vi "command_file__errors.vi"() -> ()   [LabVIEW 2016]
uses:
  Instrument_Setup.vi
  Global Variables/global.vi
panel:
  in  "fehler":bool
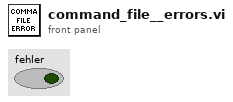
[diagram p1: front panel]
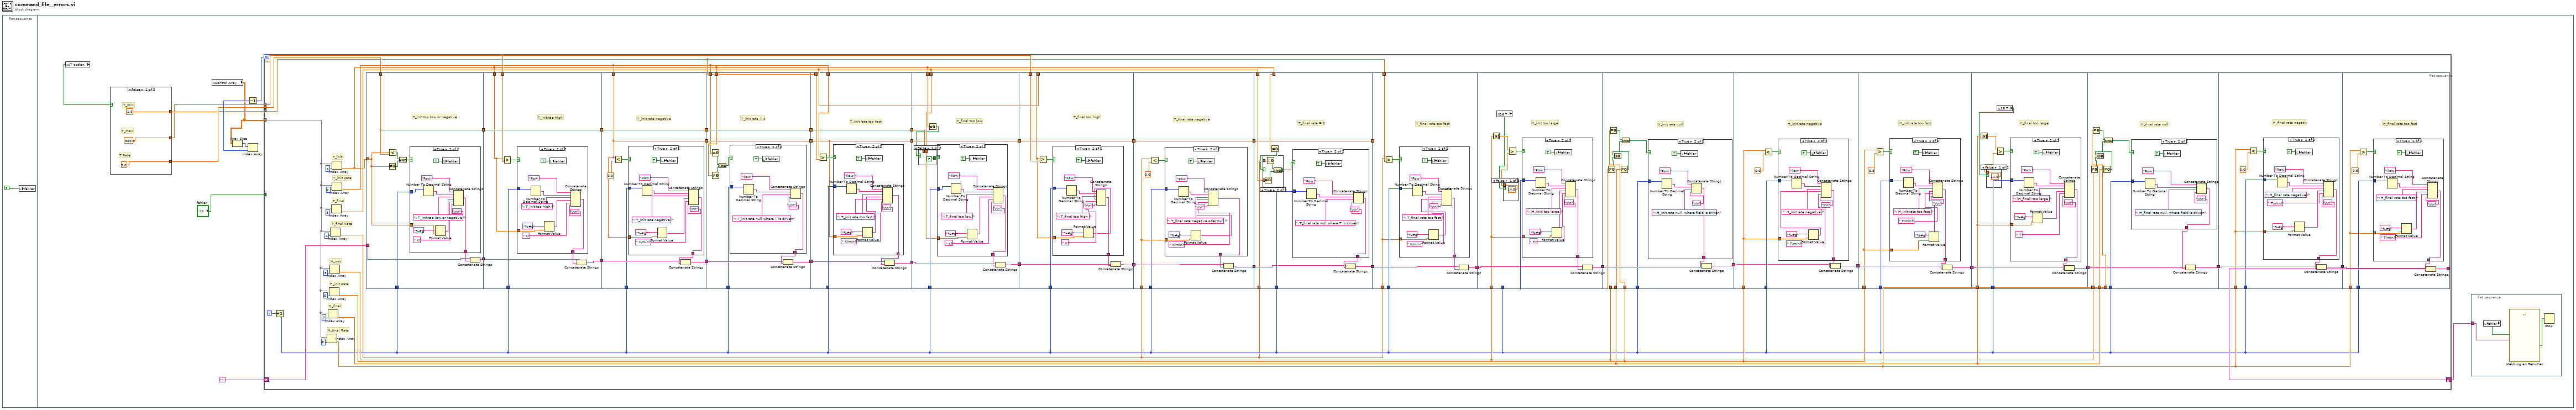
[diagram p0: block diagram]
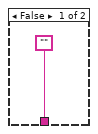
[diagram p2: hidden frame]
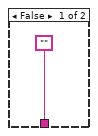
[diagram p3: hidden frame]
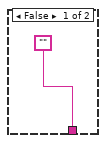
[diagram p4: hidden frame]
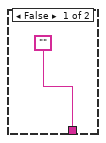
[diagram p5: hidden frame]
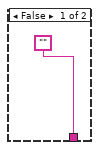
[diagram p6: hidden frame]
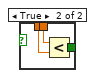
[diagram p7: hidden frame]
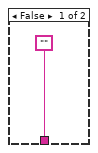
[diagram p8: hidden frame]
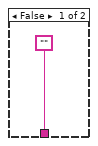
[diagram p9: hidden frame]
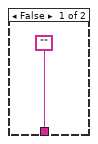
[diagram p10: hidden frame]
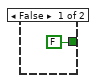
[diagram p11: hidden frame]
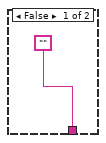
[diagram p12: hidden frame]
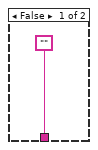
[diagram p13: hidden frame]
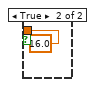
[diagram p14: hidden frame]
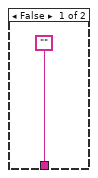
[diagram p15: hidden frame]
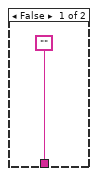
[diagram p16: hidden frame]
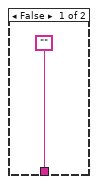
[diagram p17: hidden frame]
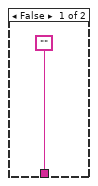
[diagram p18: hidden frame]
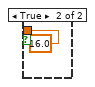
[diagram p19: hidden frame]
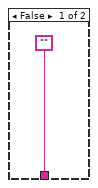
[diagram p20: hidden frame]
diagram:
  n1 = flat-sequence {
    frame #0 {
      n2 = local write "fehler"(FALSE) -> ()
    }
    frame #1 {
      n3 = global read "Instrument_Setup.vi" "JT option"() -> (w12:bool)
      n4 = case shown="False" w12 {
        tunnel: [1.6 0.02] -> w8
        tunnel: [300.0 15.0] -> w7
        tunnel: [3.0 1.0] -> w6
        frame False {
          # "T Rate"
          # "T_max"
          # "T_min"
        }
        frame True {
          # "T Rate"
          # "T_max"
          # "T_min"
        }
      }
      n5 = global read "global.vi" "Control Array"() -> (w2:dbl[][])
      n6 = Array Size(array=w2) -> (size(s)=w11:i32[])
      n7 = Index Array(array=w11) -> (element=w9:i32)  [unwired: 1 in]
      n8 = Decrement(x=w9) -> (x-1=w10:i32)
      n9 = for {
        N: w10 -> [_]
        tunnel: w2 -> [w60] mode=indexing
        tunnel: w8 -> [w59]
        tunnel: "fehler" -> [_]
        tunnel: w7 -> [w43]
        shift-right: [w35] -> w3
        shift-left: "" -> [w54]
        tunnel: w6 -> [w31]
        i -> [w57]
        # "H_final Rate"
        # "H_final"
        # "H_init Rate"
        # "H_init"
        # "T_final Rate"
        # "T_final"
        # "T_init Rate"
        # "T_init"
        n10 = Increment(x=w57) -> (x+1=w19:i32)
        n11 = Index Array(array=w60, index=8) -> (element=w32:dbl)
        n12 = Index Array(array=w60, index=7) -> (element=w34:dbl)
        n13 = Index Array(array=w60, index=6) -> (element=w40:dbl)
        n14 = Index Array(array=w60, index=5) -> (element=w33:dbl)
        n15 = Index Array(array=w60, index=4) -> (element=w18:dbl)
        n16 = Index Array(array=w60, index=3) -> (element=w17:dbl)
        n17 = Index Array(array=w60, index=1) -> (element=w16:dbl)
        n18 = Index Array(array=w60, index=2) -> (element=w20:dbl)
        n19 = flat-sequence {
          tunnel: w16 -> [w69]
          tunnel: w59 -> [w73]
          tunnel: w54 -> [w76]
          tunnel: [w75] -> w58
          tunnel: w19 -> [w74]
          tunnel: [w73] -> w47
          tunnel: w43 -> [w96]
          tunnel: w16 -> [w90]
          tunnel: w19 -> [w95]
          tunnel: w58 -> [w94]
          tunnel: [w92] -> w56
          tunnel: [w91] -> w48
          tunnel: w47 -> [w91]
          tunnel: w56 -> [w115]
          tunnel: w20 -> [w110]
          tunnel: w19 -> [w111]
          tunnel: [w113] -> w30
          tunnel: [w112] -> w28
          tunnel: w48 -> [w112]
          tunnel: [w110] -> w26
          tunnel: w30 -> [w136]
          tunnel: [w137] -> w29
          tunnel: w28 -> [w140]
          tunnel: [w140] -> w27
          tunnel: w26 -> [w139]
          tunnel: [w139] -> w25
          tunnel: w19 -> [w135]
          tunnel: w20 -> [w130]
          tunnel: w16 -> [w131]
          tunnel: [w154] -> w55
          tunnel: w20 -> [w151]
          tunnel: w19 -> [w156]
          tunnel: w29 -> [w155]
          tunnel: w31 -> [w152]
          tunnel: [w150] -> w49
          tunnel: w27 -> [w150]
          tunnel: [w149] -> w44
          tunnel: w25 -> [w149]
          tunnel: w55 -> [w177]
          tunnel: w19 -> [w178]
          tunnel: [w175] -> w53
          tunnel: w17 -> [w172]
          tunnel: w49 -> [w174]
          tunnel: [w173] -> w45
          tunnel: w44 -> [w173]
          tunnel: w16 -> [w171]
          tunnel: w19 -> [w202]
          tunnel: w53 -> [w201]
          tunnel: [w199] -> w52
          tunnel: [w198] -> w46
          tunnel: w45 -> [w198]
          tunnel: w17 -> [w196]
          tunnel: w43 -> [w197]
          tunnel: w19 -> [w222]
          tunnel: w52 -> [w221]
          tunnel: [w219] -> w24
          tunnel: w18 -> [w216]
          tunnel: [w217] -> w22
          tunnel: w46 -> [w217]
          tunnel: w24 -> [w241]
          tunnel: [w242] -> w23
          tunnel: w22 -> [w245]
          tunnel: [w245] -> w21
          tunnel: w19 -> [w243]
          tunnel: w18 -> [w240]
          tunnel: w17 -> [w239]
          tunnel: w16 -> [w238]
          tunnel: [w262] -> w51
          tunnel: w19 -> [w265]
          tunnel: w23 -> [w264]
          tunnel: w18 -> [w260]
          tunnel: w21 -> [_]
          tunnel: w31 -> [w261]
          tunnel: w51 -> [w284]
          tunnel: [w283] -> w50
          tunnel: w33 -> [w281]
          tunnel: w19 -> [w285]
          tunnel: w50 -> [w312]
          tunnel: [w311] -> w42
          tunnel: w19 -> [w310]
          tunnel: w33 -> [w309]
          tunnel: w34 -> [w308]
          tunnel: w40 -> [w302]
          tunnel: w42 -> [w324]
          tunnel: w19 -> [w325]
          tunnel: [w323] -> w41
          tunnel: w40 -> [w322]
          tunnel: [w342] -> w39
          tunnel: w19 -> [w344]
          tunnel: w41 -> [w343]
          tunnel: w40 -> [w341]
          tunnel: w39 -> [w364]
          tunnel: [w363] -> w38
          tunnel: w34 -> [w362]
          tunnel: w19 -> [w365]
          tunnel: w38 -> [w384]
          tunnel: [w383] -> w37
          tunnel: w19 -> [w388]
          tunnel: w34 -> [w387]
          tunnel: w33 -> [w386]
          tunnel: w32 -> [w385]
          tunnel: w37 -> [w405]
          tunnel: w19 -> [w406]
          tunnel: [w404] -> w36
          tunnel: w32 -> [w403]
          tunnel: [w424] -> w35
          tunnel: w36 -> [w425]
          tunnel: w19 -> [w423]
          tunnel: w32 -> [w422]
          frame #0 {
            # "T_init too low or negative"
            n20 = Not Equal To 0?(x=w69) -> (x != 0?=w72:bool)
            n21 = Less?(x=w69, y=w73) -> (x < y?=w71:bool)
            n22 = And(x=w71, y=w72) -> (x .and. y?=w70:bool)
            n23 = case shown="True" w70 {
              tunnel: w74 -> [_ w86]
              tunnel: ["" w84] -> w77
              tunnel: w69 -> [_ w81]
              frame False {
              }
              frame True {
                n24 = Number To Decimal String(number=w86) -> (decimal integer string=w85:string)  [unwired: 1 in]
                n25 = Format Value(format string="%#g", value (0)=w81) -> (output string=w79:string)  [unwired: 1 in]
                n26 = local write "fehler"(TRUE) -> ()
                n27 = Concatenate Strings("Row ", w85, ": T_init too low or negative (", w79, " K)", "\r\n") -> (w84:string)
              }
            }
            n28 = Concatenate Strings(w76, w77) -> (w75:string)
          }
          frame #1 {
            # "T_init too high"
            n29 = Greater?(x=w90, y=w96) -> (0:w97:bool)
            n30 = case shown="True" w97 {
              tunnel: ["" w105] -> w93
              tunnel: w95 -> [_ w104]
              tunnel: w90 -> [_ w99]
              frame False {
              }
              frame True {
                n31 = Number To Decimal String(number=w104) -> (decimal integer string=w106:string)  [unwired: 1 in]
                n32 = Format Value(format string="%#g", value (0)=w99) -> (output string=w101:string)  [unwired: 1 in]
                n33 = local write "fehler"(TRUE) -> ()
                n34 = Concatenate Strings("Row ", w106, ": T_init too high (", w101, " K)", "\r\n") -> (w105:string)
              }
            }
            n35 = Concatenate Strings(w94, w93) -> (w92:string)
          }
          frame #2 {
            # "T_init rate negative"
            n36 = Less?(x=w110, y=0.0) -> (x < y?=w117:bool)
            n37 = case shown="True" w117 {
              tunnel: ["" w125] -> w114
              tunnel: w111 -> [_ w124]
              tunnel: w110 -> [_ w119]
              frame False {
              }
              frame True {
                n38 = Number To Decimal String(number=w124) -> (decimal integer string=w126:string)  [unwired: 1 in]
                n39 = Format Value(format string="%#g", value (0)=w119) -> (output string=w120:string)  [unwired: 1 in]
                n40 = local write "fehler"(TRUE) -> ()
                n41 = Concatenate Strings("Row ", w126, ": T_init rate negative (", w120, " K/min)", "\r\n") -> (w125:string)
              }
            }
            n42 = Concatenate Strings(w115, w114) -> (w113:string)
          }
          frame #3 {
            # "T_init rate = 0"
            n43 = Equal To 0?(x=w130) -> (x = 0?=w133:bool)
            n44 = Not Equal To 0?(x=w131) -> (x != 0?=w134:bool)
            n45 = And(x=w133, y=w134) -> (x .and. y?=w132:bool)
            n46 = case shown="True" w132 {
              tunnel: ["" w144] -> w138
              tunnel: w135 -> [_ w143]
              frame False {
              }
              frame True {
                n47 = Number To Decimal String(number=w143) -> (decimal integer string=w145:string)  [unwired: 1 in]
                n48 = local write "fehler"(TRUE) -> ()
                n49 = Concatenate Strings("Row ", w145, ": T_init rate null where T is driven", "\r\n") -> (w144:string)
              }
            }
            n50 = Concatenate Strings(w136, w138) -> (w137:string)
          }
          frame #4 {
            # "T_init rate too fast"
            n51 = Greater?(x=w151, y=w152) -> (0:w157:bool)
            n52 = case shown="True" w157 {
              tunnel: ["" w165] -> w153
              tunnel: w156 -> [_ w164]
              tunnel: w149 -> [_ w159]
              frame False {
              }
              frame True {
                n53 = Number To Decimal String(number=w164) -> (decimal integer string=w166:string)  [unwired: 1 in]
                n54 = Format Value(format string="%#g", value (0)=w159) -> (output string=w160:string)  [unwired: 1 in]
                n55 = local write "fehler"(TRUE) -> ()
                n56 = Concatenate Strings("Row ", w166, ": T_init rate too fast (", w160, " K/min)", "\r\n") -> (w165:string)
              }
            }
            n57 = Concatenate Strings(w155, w153) -> (w154:string)
          }
          frame #5 {
            # "T_final too low"
            n58 = Not Equal To 0?(x=w171) -> (x != 0?=w170:bool)
            n59 = case shown="False" w170 {
              tunnel: [FALSE w183] -> w179
              tunnel: w174 -> [_ w182]
              tunnel: w172 -> [_ w181]
              frame False {
              }
              frame True {
                n60 = Less?(x=w181, y=w182) -> (x < y?=w183:bool)
              }
            }
            n61 = case shown="True" w179 {
              tunnel: w178 -> [_ w193]
              tunnel: ["" w191] -> w176
              tunnel: w172 -> [_ w185]
              frame False {
              }
              frame True {
                n62 = Number To Decimal String(number=w193) -> (decimal integer string=w192:string)  [unwired: 1 in]
                n63 = Format Value(format string="%#g", value (0)=w185) -> (output string=w186:string)  [unwired: 1 in]
                n64 = local write "fehler"(TRUE) -> ()
                n65 = Concatenate Strings("Row ", w192, ": T_final too low (", w186, " K)", "\r\n") -> (w191:string)
              }
            }
            n66 = Concatenate Strings(w177, w176) -> (w175:string)
          }
          frame #6 {
            # "T_final too high"
            n67 = Greater?(x=w196, y=w197) -> (0:w203:bool)
            n68 = case shown="True" w203 {
              tunnel: ["" w211] -> w200
              tunnel: w202 -> [_ w210]
              tunnel: w196 -> [_ w205]
              frame False {
              }
              frame True {
                n69 = Number To Decimal String(number=w210) -> (decimal integer string=w212:string)  [unwired: 1 in]
                n70 = Format Value(format string="%#g", value (0)=w205) -> (output string=w206:string)  [unwired: 1 in]
                n71 = local write "fehler"(TRUE) -> ()
                n72 = Concatenate Strings("Row ", w212, ": T_final too high (", w206, " K)", "\r\n") -> (w211:string)
              }
            }
            n73 = Concatenate Strings(w201, w200) -> (w199:string)
          }
          frame #7 {
            # "T_final rate negative"
            n74 = Less?(x=w216, y=0.0) -> (x < y?=w223:bool)
            n75 = case shown="True" w223 {
              tunnel: ["" w231] -> w220
              tunnel: w222 -> [_ w230]
              tunnel: w216 -> [_ w225]
              frame False {
              }
              frame True {
                n76 = Number To Decimal String(number=w230) -> (decimal integer string=w232:string)  [unwired: 1 in]
                n77 = Format Value(format string="%#g", value (0)=w225) -> (output string=w226:string)  [unwired: 1 in]
                n78 = local write "fehler"(TRUE) -> ()
                n79 = Concatenate Strings("Row ", w232, ": T_final rate negative oder null (", w226, " K/min)", "\r\n") -> (w231:string)
              }
            }
            n80 = Concatenate Strings(w221, w220) -> (w219:string)
          }
          frame #8 {
            # "T_final rate = 0"
            n81 = Not Equal To 0?(x=w238) -> (x != 0?=w237:bool)
            n82 = case shown="True" w237 {
              tunnel: w240 -> [_ w249]
              tunnel: w239 -> [_ w248]
              tunnel: [FALSE w247] -> w236
              frame False {
              }
              frame True {
                n83 = Not Equal To 0?(x=w248) -> (x != 0?=w250:bool)
                n84 = Equal To 0?(x=w249) -> (x = 0?=w251:bool)
                n85 = And(x=w251, y=w250) -> (x .and. y?=w247:bool)
              }
            }
            n86 = case shown="True" w236 {
              tunnel: ["" w255] -> w244
              tunnel: w243 -> [_ w254]
              frame False {
              }
              frame True {
                n87 = Number To Decimal String(number=w254) -> (decimal integer string=w256:string)  [unwired: 1 in]
                n88 = local write "fehler"(TRUE) -> ()
                n89 = Concatenate Strings("Row ", w256, ": T_final rate null where T is driven", "\r\n") -> (w255:string)
              }
            }
            n90 = Concatenate Strings(w241, w244) -> (w242:string)
          }
          frame #9 {
            # "T_final rate too fast"
            n91 = Greater?(x=w260, y=w261) -> (0:w266:bool)
            n92 = case shown="True" w266 {
              tunnel: ["" w274] -> w263
              tunnel: w265 -> [_ w273]
              tunnel: w260 -> [_ w268]
              frame False {
              }
              frame True {
                n93 = Number To Decimal String(number=w273) -> (decimal integer string=w275:string)  [unwired: 1 in]
                n94 = Format Value(format string="%#g", value (0)=w268) -> (output string=w269:string)  [unwired: 1 in]
                n95 = local write "fehler"(TRUE) -> ()
                n96 = Concatenate Strings("Row ", w275, ": T_final rate too fast (", w269, " K/min)", "\r\n") -> (w274:string)
              }
            }
            n97 = Concatenate Strings(w264, w263) -> (w262:string)
          }
          frame #10 {
            # "H_init too large"
            n98 = Absolute Value(x=w281) -> (abs(x)=w286:dbl)
            n99 = global read "Instrument_Setup.vi" "16 T"() -> (w280:bool)
            n100 = case shown="False" w280 {
              tunnel: [14.0 16.0] -> w279
              frame False {
              }
              frame True {
              }
            }
            n101 = Greater?(x=w286, y=w279) -> (0:w287:bool)
            n102 = case shown="True" w287 {
              tunnel: ["" w297] -> w282
              tunnel: w285 -> [_ w296]
              tunnel: w281 -> [_ w293]
              frame False {
              }
              frame True {
                n103 = Number To Decimal String(number=w296) -> (decimal integer string=w298:string)  [unwired: 1 in]
                n104 = Format Value(format string="%#g", value (0)=w293) -> (output string=w292:string)  [unwired: 1 in]
                n105 = local write "fehler"(TRUE) -> ()
                n106 = Concatenate Strings("Row ", w298, ": |H_init| too large (", w292, " T)", "\r\n") -> (w297:string)
              }
            }
            n107 = Concatenate Strings(w284, w282) -> (w283:string)
          }
          frame #11 {
            # "H_init rate null"
            n108 = Not Equal To 0?(x=w309) -> (x != 0?=w307:bool)
            n109 = Equal To 0?(x=w302) -> (x = 0?=w305:bool)
            n110 = Not Equal To 0?(x=w308) -> (x != 0?=w306:bool)
            n111 = Or(x=w306, y=w307) -> (x .or. y?=w304:bool)
            n112 = And(x=w305, y=w304) -> (x .and. y?=w303:bool)
            n113 = case shown="True" w303 {
              tunnel: ["" w317] -> w313
              tunnel: w310 -> [_ w316]
              frame False {
              }
              frame True {
                n114 = Number To Decimal String(number=w316) -> (decimal integer string=w318:string)  [unwired: 1 in]
                n115 = local write "fehler"(TRUE) -> ()
                n116 = Concatenate Strings("Row ", w318, ": H_init rate null, where field is driven", "\r\n") -> (w317:string)
              }
            }
            n117 = Concatenate Strings(w312, w313) -> (w311:string)
          }
          frame #12 {
            # "H_init rate negative"
            n118 = Less?(x=w322, y=0.0) -> (x < y?=w328:bool)
            n119 = case shown="True" w328 {
              tunnel: ["" w336] -> w326
              tunnel: w325 -> [_ w335]
              tunnel: w322 -> [_ w330]
              frame False {
              }
              frame True {
                n120 = Number To Decimal String(number=w335) -> (decimal integer string=w337:string)  [unwired: 1 in]
                n121 = Format Value(format string="%#g", value (0)=w330) -> (output string=w331:string)  [unwired: 1 in]
                n122 = local write "fehler"(TRUE) -> ()
                n123 = Concatenate Strings("Row ", w337, ": H_init rate negative (", w331, " T/min)", "\r\n") -> (w336:string)
              }
            }
            n124 = Concatenate Strings(w324, w326) -> (w323:string)
          }
          frame #13 {
            # "H_init rate too fast"
            n125 = Greater?(x=w341, y=0.5) -> (0:w345:bool)
            n126 = case shown="True" w345 {
              tunnel: ["" w355] -> w347
              tunnel: w344 -> [_ w354]
              tunnel: w341 -> [_ w349]
              frame False {
              }
              frame True {
                n127 = Number To Decimal String(number=w354) -> (decimal integer string=w356:string)  [unwired: 1 in]
                n128 = local write "fehler"(TRUE) -> ()
                n129 = Format Value(format string="%#g", value (0)=w349) -> (output string=w351:string)  [unwired: 1 in]
                n130 = Concatenate Strings("Row ", w356, ": H_init rate too fast (", w351, " T/min)", "\r\n") -> (w355:string)
              }
            }
            n131 = Concatenate Strings(w343, w347) -> (w342:string)
          }
          frame #14 {
            # "H_final too large"
            n132 = Absolute Value(x=w362) -> (abs(x)=w367:dbl)
            n133 = global read "Instrument_Setup.vi" "16 T"() -> (w360:bool)
            n134 = case shown="False" w360 {
              tunnel: [14.0 16.0] -> w361
              frame False {
              }
              frame True {
              }
            }
            n135 = Greater?(x=w367, y=w361) -> (0:w368:bool)
            n136 = case shown="True" w368 {
              tunnel: ["" w378] -> w366
              tunnel: w365 -> [_ w377]
              tunnel: w362 -> [_ w372]
              frame False {
              }
              frame True {
                n137 = Number To Decimal String(number=w377) -> (decimal integer string=w379:string)  [unwired: 1 in]
                n138 = Format Value(format string="%#g", value (0)=w372) -> (output string=w373:string)  [unwired: 1 in]
                n139 = local write "fehler"(TRUE) -> ()
                n140 = Concatenate Strings("Row ", w379, ": |H_final| too large (", w373, " T)", "\r\n") -> (w378:string)
              }
            }
            n141 = Concatenate Strings(w364, w366) -> (w363:string)
          }
          frame #15 {
            # "H_final rate null"
            n142 = Not Equal To 0?(x=w386) -> (x != 0?=w393:bool)
            n143 = Equal To 0?(x=w385) -> (x = 0?=w391:bool)
            n144 = Not Equal To 0?(x=w387) -> (x != 0?=w392:bool)
            n145 = Or(x=w392, y=w393) -> (x .or. y?=w390:bool)
            n146 = And(x=w391, y=w390) -> (x .and. y?=w389:bool)
            n147 = case shown="True" w389 {
              tunnel: ["" w398] -> w394
              tunnel: w388 -> [_ w397]
              frame False {
              }
              frame True {
                n148 = Number To Decimal String(number=w397) -> (decimal integer string=w399:string)  [unwired: 1 in]
                n149 = local write "fehler"(TRUE) -> ()
                n150 = Concatenate Strings("Row ", w399, ": H_final rate null, where field is driven", "\r\n") -> (w398:string)
              }
            }
            n151 = Concatenate Strings(w384, w394) -> (w383:string)
          }
          frame #16 {
            # "H_final rate negativ"
            n152 = Less?(x=w403, y=0.0) -> (x < y?=w409:bool)
            n153 = case shown="True" w409 {
              tunnel: ["" w417] -> w407
              tunnel: w406 -> [_ w416]
              tunnel: w403 -> [_ w413]
              frame False {
              }
              frame True {
                n154 = Number To Decimal String(number=w416) -> (decimal integer string=w418:string)  [unwired: 1 in]
                n155 = Format Value(format string="%#g", value (0)=w413) -> (output string=w412:string)  [unwired: 1 in]
                n156 = local write "fehler"(TRUE) -> ()
                n157 = Concatenate Strings("Row ", w418, ": H_final rate negative (", w412, " T/min)", "\r\n") -> (w417:string)
              }
            }
            n158 = Concatenate Strings(w405, w407) -> (w404:string)
          }
          frame #17 {
            # "H_final rate too fast"
            n159 = Greater?(x=w422, y=0.5) -> (0:w426:bool)
            n160 = case shown="True" w426 {
              tunnel: ["" w436] -> w428
              tunnel: w423 -> [_ w435]
              tunnel: w422 -> [_ w433]
              frame False {
              }
              frame True {
                n161 = Number To Decimal String(number=w435) -> (decimal integer string=w437:string)  [unwired: 1 in]
                n162 = Format Value(format string="%#g", value (0)=w433) -> (output string=w430:string)  [unwired: 1 in]
                n163 = local write "fehler"(TRUE) -> ()
                n164 = Concatenate Strings("Row ", w437, ": H_final rate too fast (", w430, " T/min)", "\r\n") -> (w436:string)
              }
            }
            n165 = Concatenate Strings(w425, w428) -> (w424:string)
          }
        }
      }
      n166 = flat-sequence {
        tunnel: w3 -> [w14]
        frame #0 {
          n167 = local read "fehler"() -> (w15:bool)
          n168 = call "Meldung an Benutzer"("Enable"=w15, "Message"=w14) -> ("OK"=w13:bool)  [unwired: 8 in, 1 out]
          n169 = Stop(stop? (T)=w13) -> ()
        }
      }
    }
  }
